vi "Swipe Scroll Demo.vi"() -> ()   [LabVIEW 2020]
uses:
  Swipe Scroll Listbox Class/SwipeScrollListbox.lvclass
  C:/Program Files/National Instruments/LabVIEW 2020/vi.lib/QSI/QControls/QControl Classes/ListBox/ListBox.lvclass
panel:
  out "Selection":dbl
  in  "Modified System Lisbox":i32(listbox)
  # "Swipe enabled Scroll"
  # "Note: You will need the QControl Toolkit to run this."
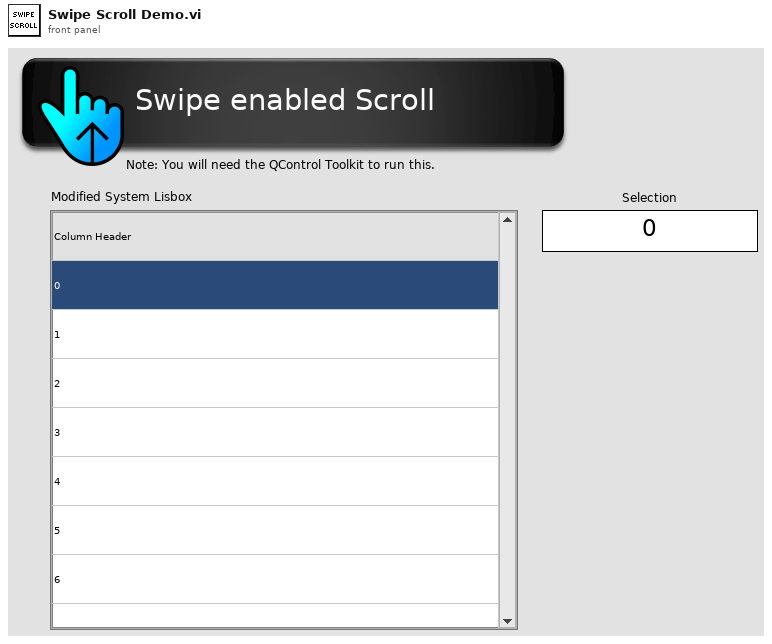
[diagram p1: front panel]
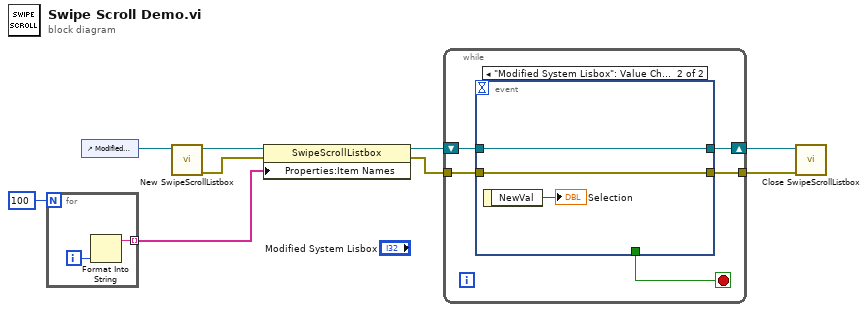
[diagram p0: block diagram]
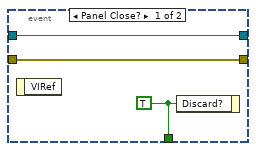
[diagram p2: hidden frame]
diagram:
  n1 = for {
    N: 100 -> [_]
    tunnel: [w11] -> w1 mode=indexing
    i -> [w10]
    n2 = Format Into String(w10) -> (resulting string=w11:string)  [unwired: 3 in, 1 out]
  }
  n3 = control-ref of="Modified System Lisbox"() -> (w6:refnum<vi>)
  n4 = call "New SwipeScrollListbox.vi"("Reference"=w6) -> ("error out"=w7:errorcluster, "SwipeScrollListbox out"=w4:refnum<class "SwipeScrollListbox.lvclass">)  [unwired: 9 in]
  n5 = property class="SwipeScrollListbox"(reference=w4, error in=w7, "Properties:Item Names"=w1) -> (reference out=w3:refnum<class "SwipeScrollListbox.lvclass">, error out=w5:errorcluster)
  n6 = while {
    shift-right: [w14] -> w9
    shift-left: w3 -> [w15]
    tunnel: w5 -> [w13]
    tunnel: [w12] -> w8
    stop <- w16 stop-if-true
    n7 = event shown="[1] \"Modified System Lisbox\": Value Change" {
      selector: _ -> [_ _]
      dyn-events: _ -> [_ _]
      timeout: _ -> [_ _]
      tunnel: [w19 _] -> w16
      tunnel: w15 -> [w18 w22]
      tunnel: [w18 w22] -> w14
      tunnel: w13 -> [w17 w21]
      tunnel: [w17 w21] -> w12
      event Panel Close? {
        w19 = TRUE ("Discard?")
        n8 = event-data() -> ()  [unwired: 1 in, 1 out]
        n9 = event-data("Discard?"=w19) -> ()  [unwired: 1 in, 1 out]
      }
      event "Modified System Lisbox": Value Change {
        n10 = event-data() -> ("NewVal"=→"Selection":i32)  [unwired: 1 in]
      }
    }
  }
  n11 = call "Close SwipeScrollListbox.vi"("error in (no error)"=w8, "SwipeScrollListbox in"=w9) -> ()  [unwired: 9 in, 1 out]
